vi "Add Tree.vi"(7 "Parent ID":string, 8 "Error In":errorcluster, 10 "Child ID":string, 11 "Tree Manager":refnum<data-value>) -> (0 "Error Out":errorcluster, 3 "Tree Manager":refnum<data-value>)   [LabVIEW 2017, in "Tree API.lvlib" / "Tree.lvclass"]
doc: "Add a Tree under a specific Parent. Both the added Tree and the Parent have to exist in the Tree Manager.\n\nIf the Tree has a parent before the new Parent replaces it. This means this method can also be used to perform a move operation."
uses:
  Tree.lvclass
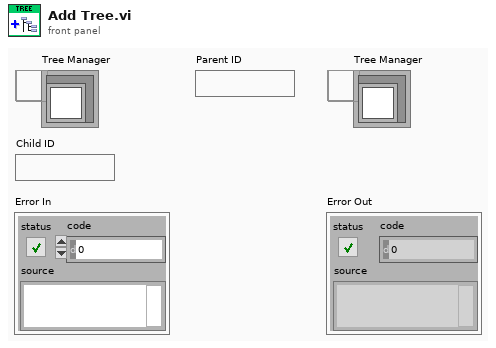
[diagram p1: front panel]
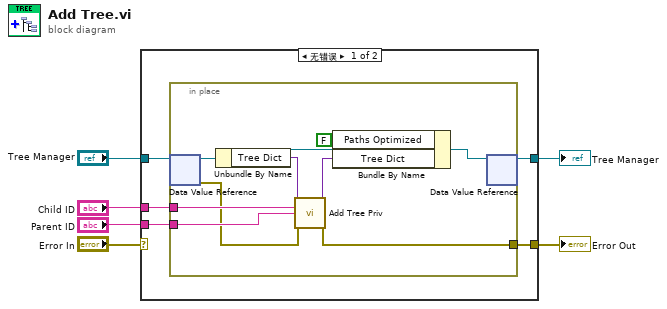
[diagram p0: block diagram]
diagram:
  n1 = case shown="无错误" "Error In" {
    selector: "Error In" -> [_ w21]
    tunnel: "Tree Manager" -> [w11 w22]
    tunnel: [w10 w22] -> w5
    tunnel: [w9 w21] -> w3
    tunnel: "Child ID" -> [w8 _]
    tunnel: "Parent ID" -> [w7 _]
    frame No Error {
      n2 = in-place {
        in-place-border: [w19] -> w9
        in-place-border: w8 -> [w17]
        in-place-border: w7 -> [w16]
        n3 = in-place-dvr #1(w11) -> (w20:refnum<class "Tree.lvclass">, w15:errorcluster)
        n4 = Unbundle By Name(w20) -> ("Tree Dict"=w14:variant)
        n5 = call "Add Tree Priv.vi"("Tree Dictionary In"=w14, "Unique ID"=w17, "Parent ID"=w16, "Error In"=w15) -> ("Tree Dictionary Out"=w13:variant, "Error Out"=w19:errorcluster)  [unwired: 10 in]
        n6 = Bundle By Name(cluster=w20, "Paths Optimized"=FALSE, "Tree Dict"=w13) -> (w18:refnum<class "Tree.lvclass">)
        n7 = in-place-dvr #1(w18) -> (w10:refnum<data-value>)  [unwired: 1 out]
      }
    }
    frame Error {
    }
  }
  "Tree Manager" <- w5
  "Error Out" <- w3
